vi "Joystick Driver Controls.vi"(7 "X":dbl, 11 "Y":dbl) -> (2 "Y":dbl, 3 "X":dbl)   [LabVIEW 2017]
uses:
  <vilib>/Rock Robotics/Network Tables/NT Read Number.vi
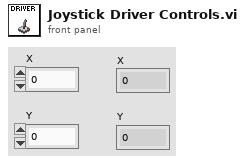
[diagram p1: front panel]
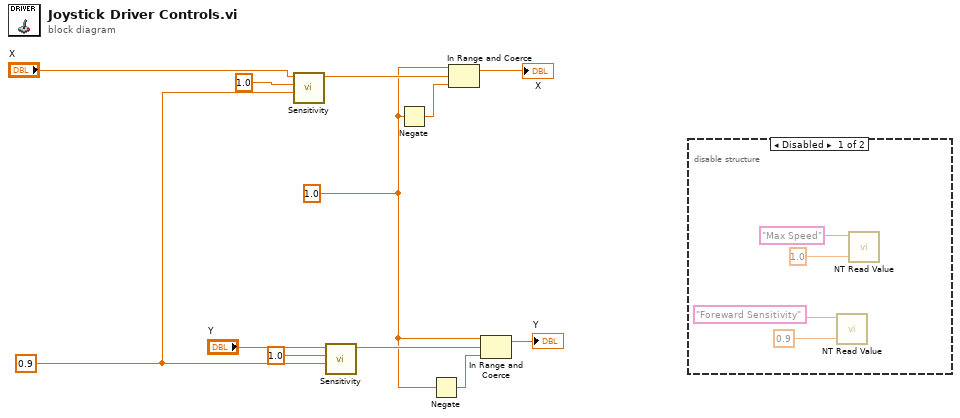
[diagram p0: block diagram]
diagram:
  w1 = 0.9
  w2 = 1.0
  n1 = call "Sensitivity.vi"("Power (z)"=w1, "Sensitivity (a)"=1.0, "Input"="X") -> ("Output"=w6:dbl)  [unwired: 8 in]
  n2 = call "Sensitivity.vi"("Power (z)"=w1, "Sensitivity (a)"=1.0, "Input"="Y") -> ("Output"=w10:dbl)  [unwired: 8 in]
  n3 = Negate(x=w2) -> (-x=w7:dbl)
  n4 = Negate(x=w2) -> (-x=w12:dbl)
  n5 = In Range and Coerce(upper limit=w2, x=w6, lower limit=w7) -> (coerced(x)=→"X":dbl)  [unwired: 1 out]
  n6 = In Range and Coerce(upper limit=w2, x=w10, lower limit=w12) -> (coerced(x)=→"Y":dbl)  [unwired: 1 out]
  n7 = disable-structure shown="Disabled" {
    frame Disabled {
      n8 = call-poly <vilib>:"NT Read Value.vi"("Default Value"=0.9, "Name"="Foreward Sensitivity") -> ()  [unwired: 8 in, 2 out]
      n9 = call-poly <vilib>:"NT Read Value.vi"("Default Value"=1.0, "Name"="Max Speed") -> ()  [unwired: 8 in, 2 out]
    }
    frame Enabled {
    }
  }
